vi "XML-RPC-LV client.vi"(8 "error in (no error)":errorcluster, 10 "method call":string="POST / HTTP/1.0\r\nContent-Type: text/xml\r\nUser-Agent: XML-RPC.NET\r\nHost: \r\nContent-Length: 125\n\n<?xml version=\"1.0\" encoding=\"UTF-8\"?>\n<methodCall>\n<methodName>StopServer</methodName>\n  <params>\n\n  </params>\n</methodCall>", 11 "Connection Parameters":T1={"address"="localhost", "remote port"=8080, "bytes to read"=100, "read timeout ms (25000)"=1000, "write (request) timeout ms (25000)"=25000}) -> (0 "error out":errorcluster, 3 "method response":string)   [LabVIEW 2009]
doc: "Open a TCP connection to an XML-RPC Server, send the method call to the server and read the method response"
uses:
  Connection Parameters.ctl
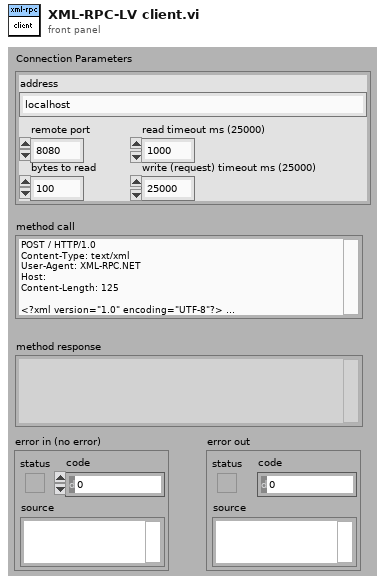
[diagram p1: front panel]
types:
  T1 = typedef "Connection Parameters.ctl" = cluster{"address":string, "remote port":u16, "bytes to read":i32, "read timeout ms (25000)":i32, "write (request) timeout ms (25000)":i32}
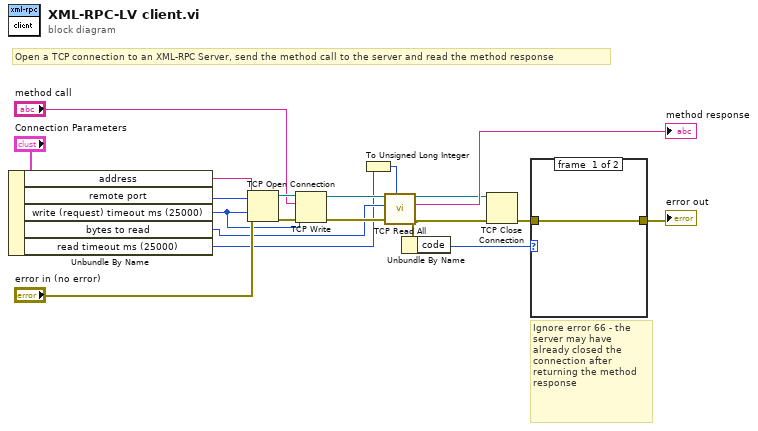
[diagram p0: block diagram]
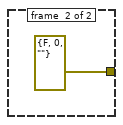
[diagram p2: hidden frame]
diagram:
  # "Ignore error 66 - the server may have already closed the connection after returning the method response"
  # "Open a TCP connection to an XML-RPC Server, send the method call to the server and read the method response"
  n1 = Unbundle By Name("Connection Parameters") -> ("address"=w12:string, "remote port"=w11:u16, "write (request) timeout ms (25000)"=w10:i32, "bytes to read"=w9:i32, "read timeout ms (25000)"=w2:i32)
  n2 = TCP Open Connection(address=w12, remote port or service name=w11, timeout ms (60000)=w10, error in (no error)="error in (no error)") -> (connection ID=w18:refnum<k5>, error out=w19:errorcluster)  [unwired: 1 in]
  n3 = TCP Write(connection ID=w18, data in="method call", error in (no error)=w19, 9:w10) -> (connection ID out=w16:refnum<k5>, error out=w17:errorcluster)  [unwired: 1 out]
  n4 = To Unsigned Long Integer(number=w2) -> (unsigned 32bit integer=w1:u32)
  n5 = call "TCP Read All.vi"("Function Timeout"=w1, "error in"=w17, "Bytes Per Loop"=w9, "connection ID in"=w16) -> ("error out"=w7:errorcluster, "data out"=→"method response":string, "connection ID out"=w4:refnum<k5>)  [unwired: 5 in]
  n6 = Unbundle By Name(w7) -> ("code"=w8:i32)
  n7 = TCP Close Connection(connection ID=w4, error in (no error)=w7) -> (error out=w6:errorcluster)  [unwired: 1 in, 1 out]
  n8 = case shown="66" w8 {
    tunnel: w6 -> [w20 _]
    tunnel: [w20 errorcluster {"status"=FALSE, "code"=0, "source"=""} ("error out")] -> w3
    frame #0 {
    }
    frame #1 {
    }
  }
  "error out" <- w3
